vi "PH_SHS_Analysis_Calibrator.allocate or free img space.vi"(0 "i ref in":refnum<vi>, 2 "Allocate?":bool, 5 "error in (no error)":errorcluster) -> (14 "i ref out":refnum<vi>, 19 "error out":errorcluster)   [LabVIEW 2014, in "PH_SHS_Analysis_Calibrator.lvlib"]
doc: "This VI is forseen to be used in constructor or destructor. If Allocate? = true is chosen, memory space for several images is allocated. If false is chosen, it is freed."
uses:
  PH_SHS_Analysis_Calibrator.lvlib
  CS_Core/CSSystem/CSSystemLib/CSSystemLib.lvlib
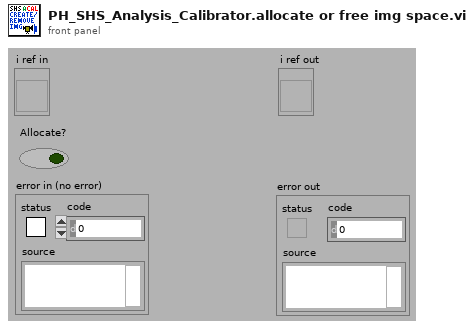
[diagram p1: front panel]
types:
  T1 = typedef "PH_SHS_Analysis_Calibrator.lvlib/PH_SHS_Analysis_Calibrator.i attribute.ctl" = cluster{"GUI Refs":cluster{"Available Cams":refnum<vi>, "OK":refnum<vi>, "Skip":refnum<vi>, "Repeat":refnum<vi>, "Cancel":refnum<vi>, "Dialog":refnum<vi>, "Enough Images?":refnum<vi>}, "Cam instances":string[], "Status":cluster{"#":i32, "Data calculated":bool, "Wanted #":i32}, "IMAQ Image Array":T2[], "Pixel Size [µm]":dbl, "MLA Pitch [µm]":dbl, "Method":enum16{"automatic", "manual"}, "Enough Images?":bool, "SHS Reference Result":T3, "Calculation Error":errorcluster}
  T2 = typedef "IMAQ Image.ctl" = refnum<image>
  T3 = typedef "SHS_Common.lvlib/SHSReference.ctl" = cluster{"Reference":T4[][], "Lens Array Pitch [px]":dbl}
  T4 = typedef "SHS_Common.lvlib/ReferencePoint.ctl" = cluster{"Rect":T5, "Point":T6}
  T5 = typedef "SHS_Common.lvlib/Rectangle.ctl" = cluster{"Left":i32, "Top":i32, "Right":i32, "Bottom":i32}
  T6 = typedef "SHS_Common.lvlib/Point.ctl" = cluster{"x":dbl, "y":dbl, "valid?":bool, "weight":dbl}
  T7 = typedef "Image Type" = u32
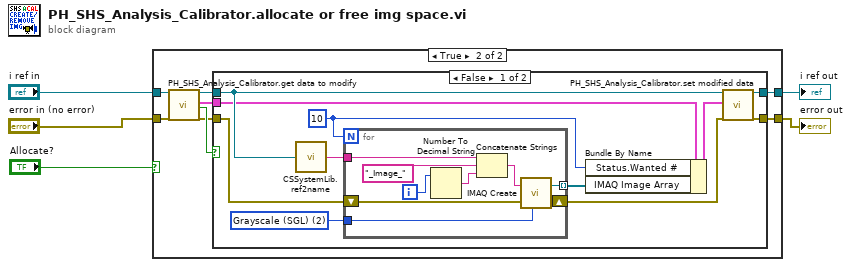
[diagram p0: block diagram]
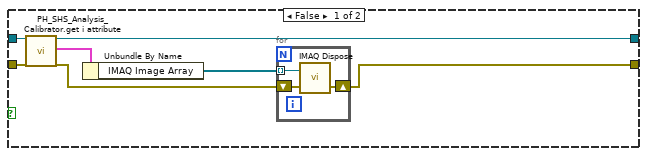
[diagram p2: hidden frame]
diagram:
  n1 = case shown="True" "Allocate?" {
    tunnel: [w7 w22] -> w5
    tunnel: [w9 w21] -> w4
    tunnel: "error in (no error)" -> [w12 w18]
    tunnel: "i ref in" -> [w11 w17]
    frame False {
      n2 = call "PH_SHS_Analysis_Calibrator.get i attribute.vi"("i ref in"=w11, "error in (no error)"=w12) -> ("i ref out"=w9:refnum<vi>, "i attribute"=w10:T1, "error out"=w8:errorcluster)  [unwired: 15 in]
      n3 = Unbundle By Name(w10) -> ("IMAQ Image Array"=w6:T2[])
      n4 = for {
        shift-right: [w14] -> w7
        shift-left: w8 -> [w15]
        tunnel: w6 -> [w13] mode=indexing
        n5 = call "IMAQ Dispose"("Image"=w13, "error in (no error)"=w15) -> ("error out"=w14:errorcluster)  [unwired: 4 in]
      }
    }
    frame True {
      n6 = call "PH_SHS_Analysis_Calibrator.get data to modify.vi"("i ref in"=w17, "error in (no error)"=w18) -> ("i ref out"=w20:refnum<vi>, "i attribute"=w16:T1, "timed out"=w23:bool, "error out"=w19:errorcluster)  [unwired: 14 in]
      n7 = case shown="False" w23 {
        tunnel: w19 -> [w27 w44]
        tunnel: w20 -> [w26 w45]
        tunnel: [w34 w45] -> w21
        tunnel: [w33 w44] -> w22
        tunnel: w16 -> [w25 _]
        frame False {
          w24 = 10
          w30 = T7 2 items=["Grayscale (U8)", "Grayscale (I16)", "Grayscale (SGL)", "Complex (CSG)", "RGB (U32)", "HSL (U32)", "RGB (U64)"] ("Image Type")
          n8 = call "CSSystemLib.ref2name.vi"("obj refnum"=w26) -> ("name"=w28:string)
          n9 = for {
            N: w24 -> [_]
            shift-right: [w43] -> w31
            shift-left: w27 -> [w42]
            tunnel: w30 -> [w41]
            tunnel: [w40] -> w29 mode=indexing
            tunnel: w28 -> [w39]
            i -> [w37]
            n10 = Number To Decimal String(number=w37) -> (decimal integer string=w36:string)  [unwired: 1 in]
            n11 = Concatenate Strings(w39, "_Image_" ("string"), w36) -> (w35:string)
            n12 = call "IMAQ Create"("Image Name"=w35, "Image Type"=w41, "error in (no error)"=w42) -> ("New Image"=w40:T2, "error out"=w43:errorcluster)  [unwired: 2 in]
          }
          n13 = Bundle By Name(cluster=w25, "Status.Wanted #"=w24, "IMAQ Image Array"=w29) -> (w32:T1)
          n14 = call "PH_SHS_Analysis_Calibrator.set modified data.vi"("i ref in"=w26, "i attribute"=w32, "error in (no error)"=w31) -> ("i ref out"=w34:refnum<vi>, "error out"=w33:errorcluster)  [unwired: 15 in]
        }
        frame True {
        }
      }
    }
  }
  "error out" <- w5
  "i ref out" <- w4
